vi "Start.vi"(8 "error in (no error)":errorcluster, 11 "Electrophysiology in":refnum<class "Electrophysiology.lvclass">) -> (0 "error out":errorcluster, 3 "Electrophysiology out":refnum<class "Electrophysiology.lvclass">)   [LabVIEW 2010, in "Electrophysiology.lvclass"]
uses:
  Electrophysiology.lvclass
  Electrophysiology.lvclass/Electrophysiology.ctl
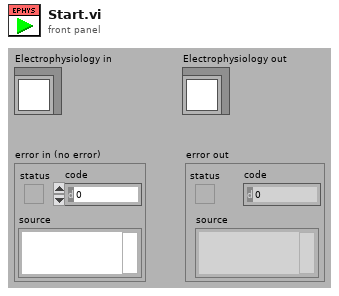
[diagram p1: front panel]
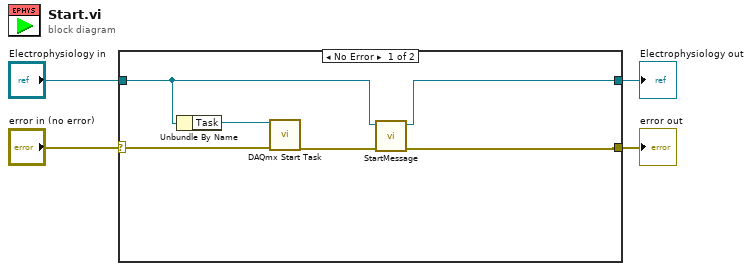
[diagram p0: block diagram]
diagram:
  n1 = case shown="No Error" "error in (no error)" {
    selector: "error in (no error)" -> [w9 w12]
    tunnel: [w7 w12] -> w3
    tunnel: [w5 w11] -> w1
    tunnel: "Electrophysiology in" -> [w6 w11]
    frame No Error {
      n2 = Unbundle By Name(w6) -> ("Task"=w10:refnum<k21>)
      n3 = call <vilib>:"DAQmx Start Task.vi"("task/channels in"=w10, "error in"=w9) -> ("error out"=w8:errorcluster)  [unwired: 12 in, 1 out]
      n4 = call-dynamic "StartMessage.vi"("error in (no error)"=w8, "AcquistionObject in"=w6) -> ("error out"=w7:errorcluster, "AcquistionObject out"=w5:refnum<class "Electrophysiology.lvclass">)  [unwired: 8 in]
    }
    frame Error {
    }
  }
  "error out" <- w3
  "Electrophysiology out" <- w1
